vi "VeriStand Framework Configuration.Get Device Reference.vi"(11 "VeriStand Framework Configuration in":refnum<class "VeriStand DSF.Framework.Configuration.lvclass">) -> (2 "Device Item Ref":T1=18446744073709551615 format="%.0x", 3 "VeriStand Framework Configuration out":refnum<class "VeriStand DSF.Framework.Configuration.lvclass">)   [LabVIEW 2017, in "Data Sharing Framework Engine.lvlib" / "VeriStand DSF.Framework.Configuration.lvclass"]
uses:
  VeriStand DSF.Framework.Configuration.lvclass
  <vilib>/NI Veristand/Custom Device API/Custom Device Item Ref.ctl
  VeriStand DSF.Framework.Configuration.lvclass/VeriStand DSF.Framework.Configuration.ctl
  <vilib>/NI Veristand/Custom Device API/Custom Device API.lvlib
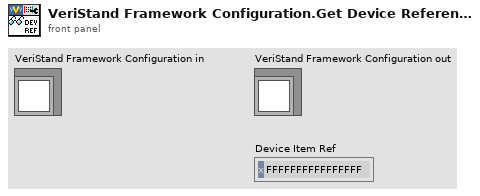
[diagram p1: front panel]
types:
  T1 = typedef "Custom Device API.lvlib/Custom Device Item Ref.ctl" = u64
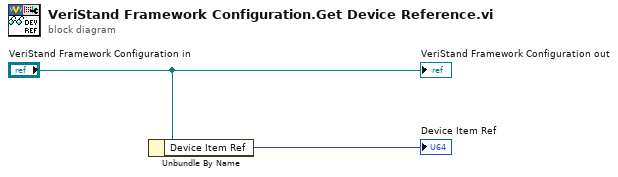
[diagram p0: block diagram]
diagram:
  n1 = Unbundle By Name("VeriStand Framework Configuration in") -> ("Device Item Ref"=→"Device Item Ref":T1)
  "VeriStand Framework Configuration out" <- "VeriStand Framework Configuration in"
